vi "DataLog Read Point At Index.vi"(0 "tag log directory":path, 7 "log index":dbl, 11 "error in (no error)":errorcluster) -> (4 "dup tag log directory":path, 8 "point":T1 {"value" format="%.3e"; "time" format="%<%H:%M:%S%2u\n%Y/%m/%d>T"}, 15 "error out":errorcluster)   [LabVIEW 2012]
doc: "Attempts to read the point at the specified index. This VI is not guaranteed to fail when indexing at or beyond the write index."
uses:
  typedefs/clusters/t_DataLog Point.ctl
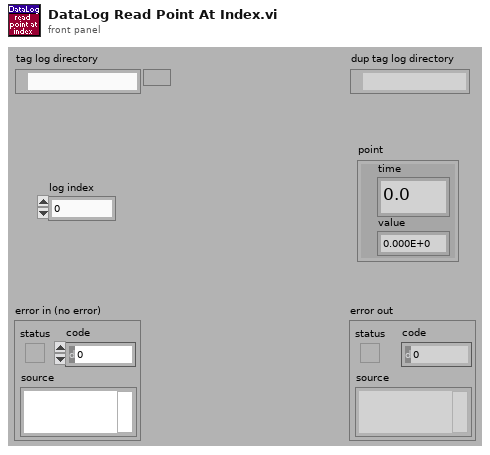
[diagram p1: front panel]
types:
  T1 = typedef "t_DataLog Point.ctl" = cluster{"time":dbl, "value":dbl}
  T2 = enum16{"deny read/write", "deny write-only", "deny none"}
  T3 = enum16{"read/write", "read-only", "write-only", "write-only (truncate)"}
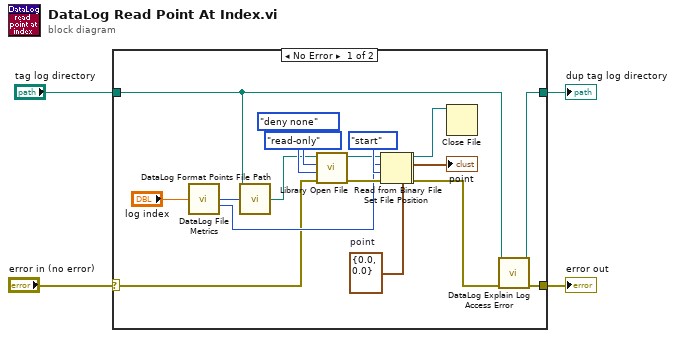
[diagram p0: block diagram]
diagram:
  n1 = case shown="No Error" "error in (no error)" {
    selector: "error in (no error)" -> [w7 w25]
    tunnel: [w11 w25] -> w4
    tunnel: "tag log directory" -> [w9 w24]
    tunnel: [w8 w24] -> w1
    frame No Error {
      w16 = T1 {"time"=0.0, "value"=0.0}  # point
      n2 = call "DataLog File Metrics.vi"("point index"="log index") -> ("log file index"=w13:i32, "log file offset"=w17:i32)  [unwired: 9 in, 4 out]
      n3 = call "DataLog Format Points File Path.vi"("tag log directory"=w9, "log file index"=w13) -> ("log file path"=w12:path)  [unwired: 12 in, 1 out]
      n4 = call "Library Open File.vi"("error in (no error)"=w7, "deny mode (deny none)"=T2."deny none" ("deny mode (2)"), "open mode (read/write)"=T3."read-only" ("open mode (0)"), "file path"=w12) -> ("error out"=w20:errorcluster, "refnum"=w19:refnum<file>)  [unwired: 2 in]
      n5 = Set File Position(offset (in bytes) (0)=w17, refnum=w19, from (0:start)=enum16{"start", "end", "current"}."start" ("pos mode (0:2)"), error in=w20) -> (refnum out=w6:refnum<file>, error out=w5:errorcluster)
      n6 = Read from Binary File(5:w16, 8:w5, 11:w6) -> (0:w10:errorcluster, 2:→"point":T1, 3:w18:refnum<file>)  [unwired: 3 in, 1 out]
      n7 = Close File(refnum=w18) -> ()  [unwired: 1 in, 2 out]
      n8 = call "DataLog Explain Log Access Error.vi"("tag log directory"=w9, "error in"=w10) -> ("dup tag log directory"=w8:path, "error out"=w11:errorcluster)  [unwired: 12 in]
    }
    frame Error {
    }
  }
  "error out" <- w4
  "dup tag log directory" <- w1
